vi "Buttons to Message.vi"(6 "Start/Stop Ref":T3, 8 "Reset":bool, 9 "Start/Stop Controls":T4, 11 "State Machine Data":T1={"Control State"="", "Status Message"="", "Speed"=0.0, "Pressure"=0.0, "Target Pressure"=0.0, "Apply Brake Ref"=refnum, "Release Brake Ref"=refnum, "Extend Ref"=refnum, "Retract Ref"=refnum, "Pressure Ref"=refnum, "Data Display Ref"=refnum, "Exit Button Ref"=refnum, "Bool"=TRUE, "Status"={"Extend"=FALSE, "Brake"=FALSE, "Retract"=FALSE}}) -> (3 "State Machine Data Out":T1={"Control State"="", "Status Message"="", "Speed"=0.0, "Pressure"=0.0, "Target Pressure"=0.0, "Apply Brake Ref"=refnum, "Release Brake Ref"=refnum, "Extend Ref"=refnum, "Retract Ref"=refnum, "Pressure Ref"=refnum, "Data Display Ref"=refnum, "Exit Button Ref"=refnum, "Bool"=TRUE, "Status"={"Extend"=FALSE, "Brake"=FALSE, "Retract"=FALSE}})   [LabVIEW 2021]
uses:
  Controls/State Machine Data.ctl
  Controls/Status Lights.ctl
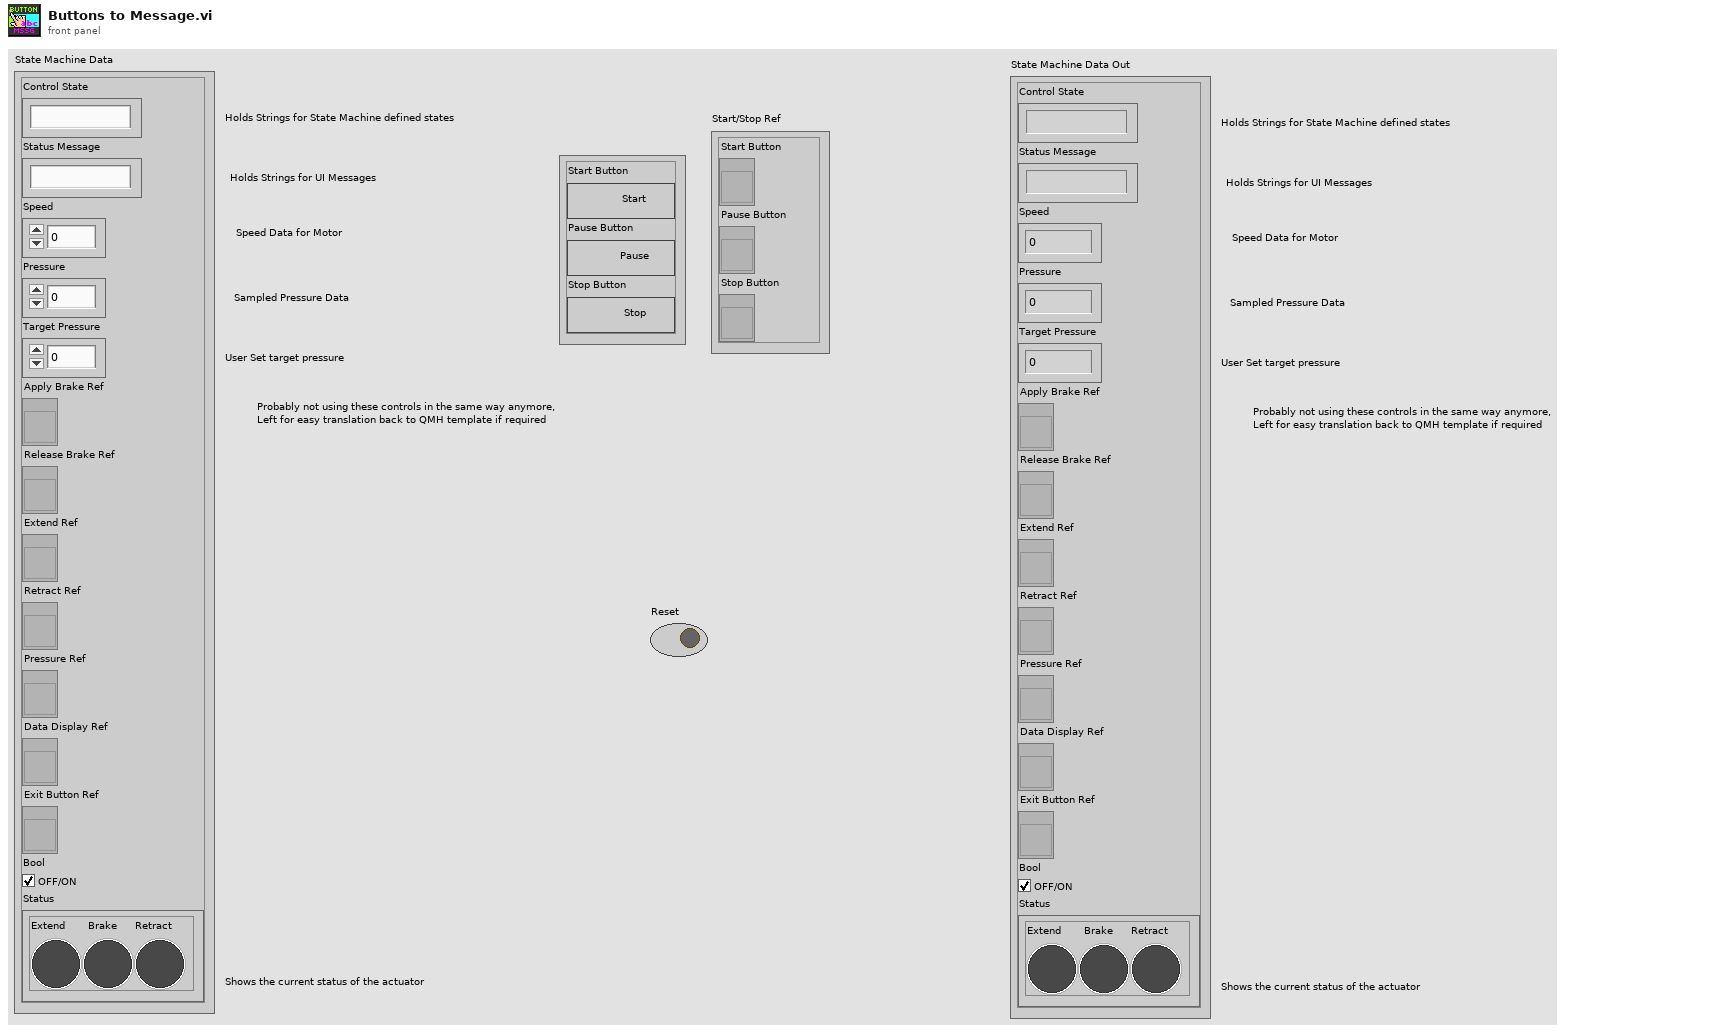
[diagram p1: front panel]
types:
  T1 = typedef "State Machine Data.ctl" = cluster{"Control State":string, "Status Message":string, "Speed":dbl, "Pressure":dbl, "Target Pressure":dbl, "Apply Brake Ref":refnum<vi>, "Release Brake Ref":refnum<vi>, "Extend Ref":refnum<vi>, "Retract Ref":refnum<vi>, "Pressure Ref":refnum<vi>, "Data Display Ref":refnum<vi>, "Exit Button Ref":refnum<vi>, "Bool":bool, "Status":T2}
  T2 = typedef "Status Lights.ctl" = cluster{"Extend":bool, "Brake":bool, "Retract":bool}
  T3 = cluster{"Start Button":refnum<vi>, "Pause Button":refnum<vi>, "Stop Button":refnum<vi>}
  T4 = cluster{"Start Button":bool, "Pause Button":bool, "Stop Button":bool}
  T5 = enum8{"Enabled", "Disabled", "Disabled and Grayed Out"}
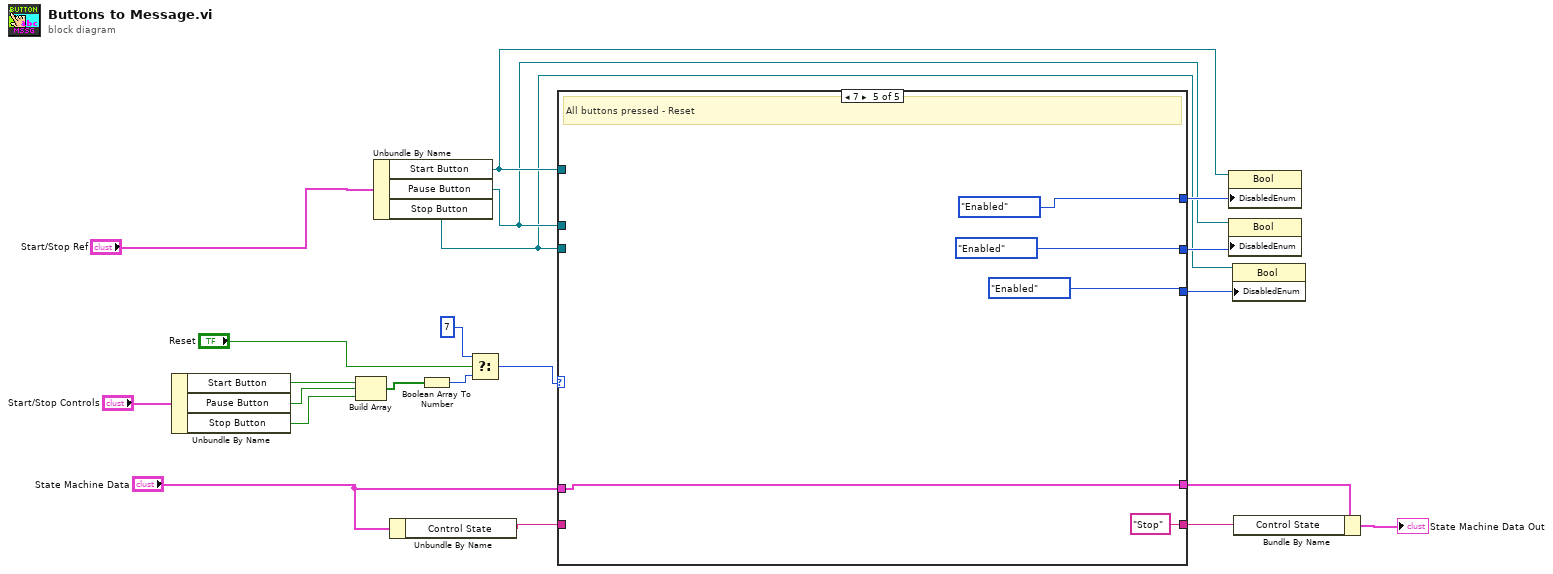
[diagram p0: block diagram]
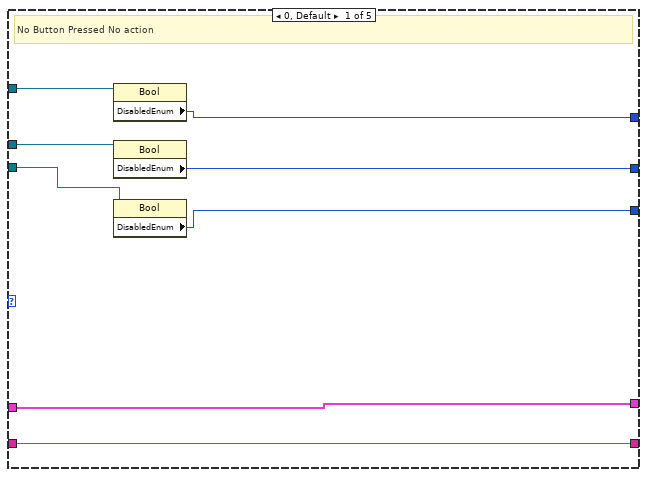
[diagram p2: hidden frame]
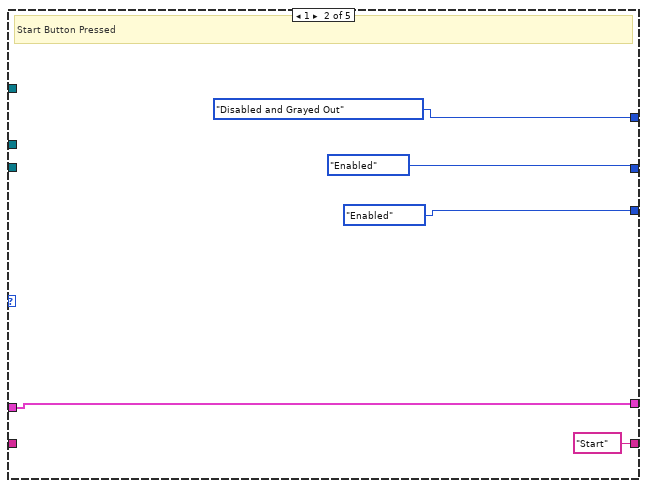
[diagram p3: hidden frame]
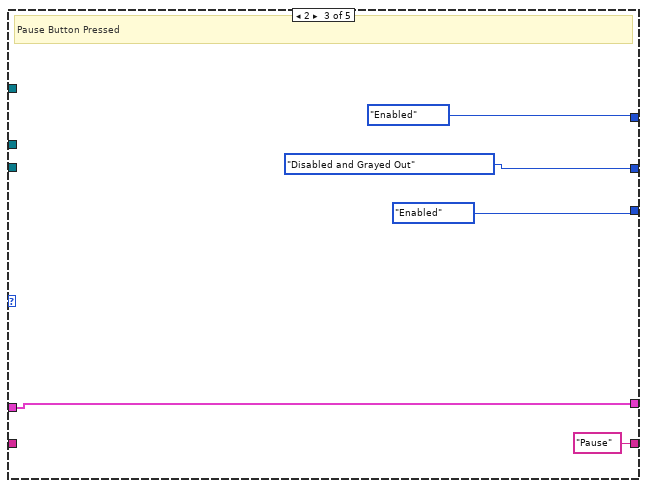
[diagram p4: hidden frame]
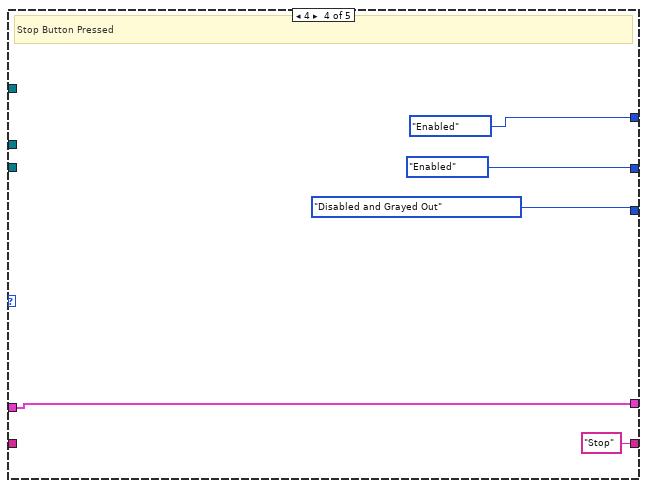
[diagram p5: hidden frame]
diagram:
  n1 = Unbundle By Name("Start/Stop Controls") -> ("Start Button"=w17:bool, "Pause Button"=w19:bool, "Stop Button"=w18:bool)
  n2 = Build Array(w17, w19, w18) -> (w20:bool[])
  n3 = Unbundle By Name("Start/Stop Ref") -> ("Start Button"=w7:refnum<vi>, "Pause Button"=w6:refnum<vi>, "Stop Button"=w5:refnum<vi>)
  n4 = Unbundle By Name("State Machine Data") -> ("Control State"=w11:string)
  n5 = Boolean Array To Number(Boolean array=w20) -> (number=w3:u32)
  n6 = Select(t=u32 7, s="Reset", f=w3) -> (s? t:f=w4:u32)
  n7 = case shown="7" w4 {
    tunnel: w6 -> [w26 _ _ _ _]
    tunnel: w5 -> [w25 _ _ _ _]
    tunnel: [w29 T5."Disabled and Grayed Out" ("Disabled") T5."Enabled" ("Disabled") T5."Enabled" ("Disabled") T5."Enabled" ("Disabled")] -> w15
    tunnel: [w28 T5."Enabled" ("Disabled") T5."Disabled and Grayed Out" ("Disabled") T5."Enabled" ("Disabled") T5."Enabled" ("Disabled")] -> w14
    tunnel: [w27 T5."Enabled" ("Disabled") T5."Enabled" ("Disabled") T5."Disabled and Grayed Out" ("Disabled") T5."Enabled" ("Disabled")] -> w13
    tunnel: [w24 w31 w35 w40 w45] -> w10
    tunnel: "State Machine Data" -> [w24 w31 w35 w40 w45]
    tunnel: [w23 "Start" ("Control State") "Pause" ("Control State") "Stop" ("Control State") "Stop" ("Control State")] -> w8
    tunnel: w11 -> [w23 _ _ _ _]
    tunnel: w7 -> [w22 _ _ _ _]
    frame 0, Default {
      # "No Button Pressed No action"
      n8 = property class="Bool"(reference=w22) -> ("DisabledEnum"=w29:T5)  [unwired: 1 in, 2 out]
      n9 = property class="Bool"(reference=w26) -> ("DisabledEnum"=w28:T5)  [unwired: 1 in, 2 out]
      n10 = property class="Bool"(reference=w25) -> ("DisabledEnum"=w27:T5)  [unwired: 1 in, 2 out]
    }
    frame 1 {
      # "Start Button Pressed"
    }
    frame 2 {
      # "Pause Button Pressed"
    }
    frame 4 {
      # "Stop Button Pressed"
    }
    frame 7 {
      # "All buttons pressed - Reset"
    }
  }
  n11 = property class="Bool"(reference=w7, "DisabledEnum"=w15) -> ()  [unwired: 1 in, 2 out]
  n12 = property class="Bool"(reference=w6, "DisabledEnum"=w14) -> ()  [unwired: 1 in, 2 out]
  n13 = property class="Bool"(reference=w5, "DisabledEnum"=w13) -> ()  [unwired: 1 in, 2 out]
  n14 = Bundle By Name(cluster=w10, "Control State"=w8) -> (→"State Machine Data Out":T1)
